vi "LibXML_AddElementsAsSibling.vi"(8 "error in":errorcluster, 9 "XML-tree":T1[](array[typedef]), 10 "node in":u32, 11 "doc":u32) -> (0 "error out":errorcluster, 1 "first written node":u32, 2 "Node-out":u32, 3 "doc copy out":u32)   [LabVIEW 2019, in "Tools.lvlib" / "LibXML.lvlib"]
doc: "Writes the XML-tree to document under the parentnode.\nThe first element of the XML-tree should contain parent=0, referring to the parentnode."
uses:
  LibXML.lvlib
  LibXML_Element.ctl
  LibXML_Attribute.ctl
panel:
  # "This software is FREE licensed under the GNU Lesser General Public License (see license.txt)."
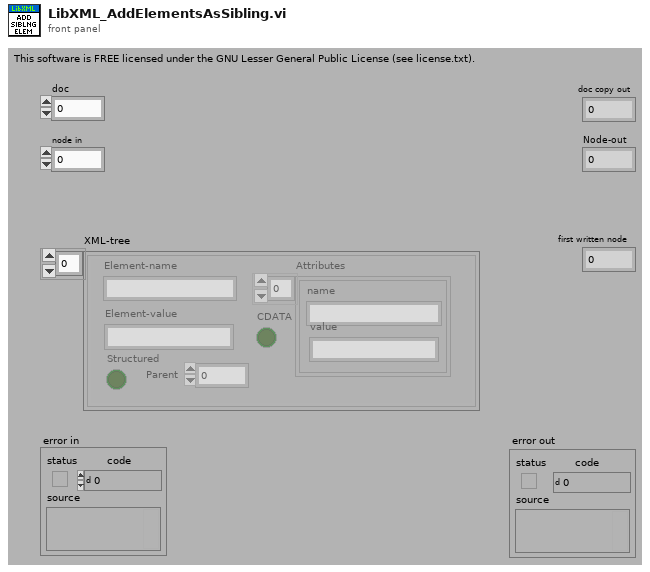
[diagram p1: front panel]
types:
  T1 = typedef "Tools.lvlib/LibXML.lvlib/LibXML_Element.ctl" = cluster{"Element-name":string, "Attributes":T2[], "Element-value":string, "CDATA":bool, "Parent":i32, "Structured":bool}
  T2 = typedef "Tools.lvlib/LibXML.lvlib/LibXML_Attribute.ctl" = cluster{"name":string, "value":string}
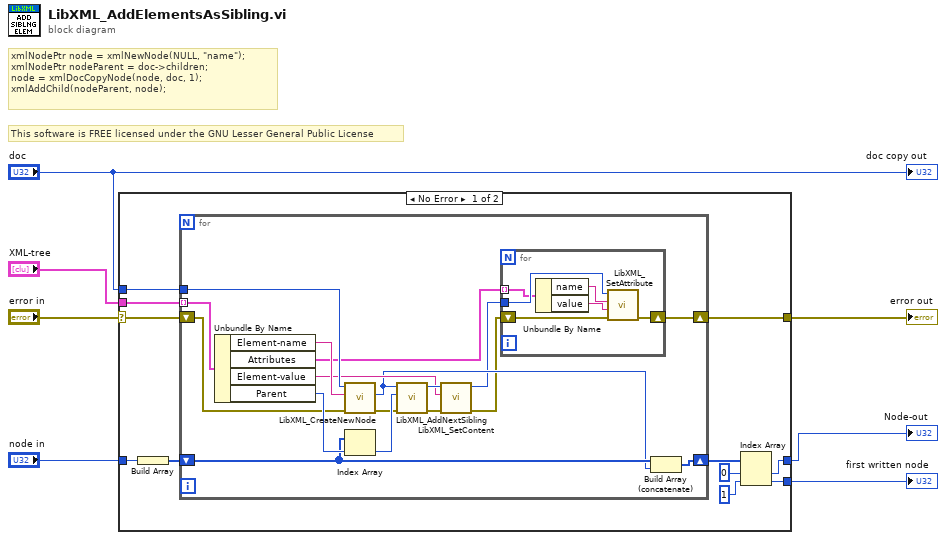
[diagram p0: block diagram]
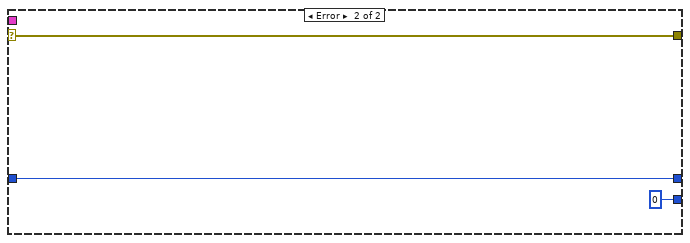
[diagram p2: hidden frame]
diagram:
  # "xmlNodePtr node = xmlNewNode(NULL, \"name\");\nxmlNodePtr nodeParent = doc->children;\nnode = xmlDocCopyNode(node, doc, 1);\nxmlAddChild(nodeParent, node);"
  # "This software is FREE licensed under the GNU Lesser General Public License"
  n1 = case shown="No Error" "error in" {
    selector: "error in" -> [w15 w43]
    tunnel: [w18 w43] -> w7
    tunnel: "doc" -> [w14 _]
    tunnel: "node in" -> [w13 w44]
    tunnel: [w11 w44] -> w4
    tunnel: [w9 u32 0 ("node in")] -> w2
    tunnel: "XML-tree" -> [w8 _]
    frame No Error {
      n2 = Build Array(w13) -> (w12:u32[])
      n3 = for {
        tunnel: w8 -> [w35] mode=indexing
        shift-right: [w20] -> w18
        shift-left: w15 -> [w23]
        tunnel: w14 -> [w34]
        shift-right: [w25] -> w10
        shift-left: w12 -> [w28]
        n4 = Unbundle By Name(w35) -> ("Element-name"=w33:string, "Attributes"=w19:T2[], "Element-value"=w29:string, "Parent"=w32:i32)
        n5 = call "LibXML_CreateNewNode.vi"("error in"=w23, "name"=w33, "doc"=w34) -> ("error out"=w24:errorcluster, "nodePtr out"=w27:u32)  [unwired: 6 in, 1 out]
        n6 = Index Array(array=w28, index=w32) -> (element=w31:u32)
        n7 = call "LibXML_AddNextSibling.vi"("error in"=w24, "sibling node"=w31, "new node"=w27) -> ("error out"=w22:errorcluster, "node copy"=w30:u32)  [unwired: 7 in]
        n8 = call "LibXML_SetContent.vi"("error in (no error)"=w22, "content"=w29, "node"=w30) -> ("error out"=w21:errorcluster, "node copy"=w26:u32)  [unwired: 7 in]
        n9 = for {
          tunnel: w26 -> [w41]
          tunnel: w19 -> [w40] mode=indexing
          shift-right: [w36] -> w20
          shift-left: w21 -> [w37]
          n10 = Unbundle By Name(w40) -> ("name"=w39:string, "value"=w38:string)
          n11 = call "LibXML_SetAttribute.vi"("error in"=w37, "value"=w38, "name"=w39, "node"=w41) -> ("error out"=w36:errorcluster)  [unwired: 6 in, 1 out]
        }
        n12 = Build Array (concatenate)(w28, w27) -> (w25:u32[])
      }
      n13 = Index Array(array=w10, index #1=0 ("Index"), index #2=1 ("Index")) -> (element #1=w11:u32, element #2=w9:u32)
    }
    frame Error {
    }
  }
  "error out" <- w7
  "Node-out" <- w4
  "first written node" <- w2
  "doc copy out" <- "doc"
